vi "strip highlighting.vi"(0 "input string":string) -> (2 "Selection":bool, 3 "Selection cluster":cluster{i32, i32, "selected string":string}, 4 "output string":string, 6 "Highlighted string":string, 8 "Highlighting":bool, 10 "Line #":i32, 15 "error out":errorcluster)   [LabVIEW 2018]
uses:
  <vilib>/regexp/Match Regular Expression.xnode
panel:
  out "whole match":string
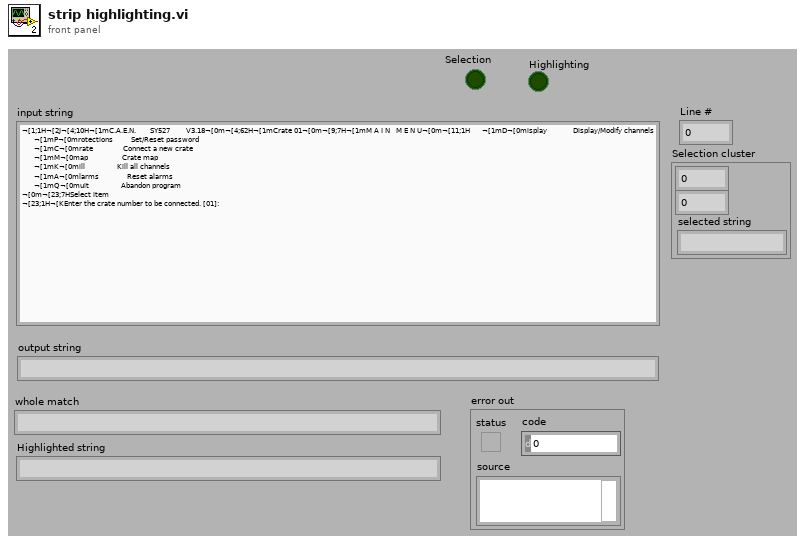
[diagram p1: front panel]
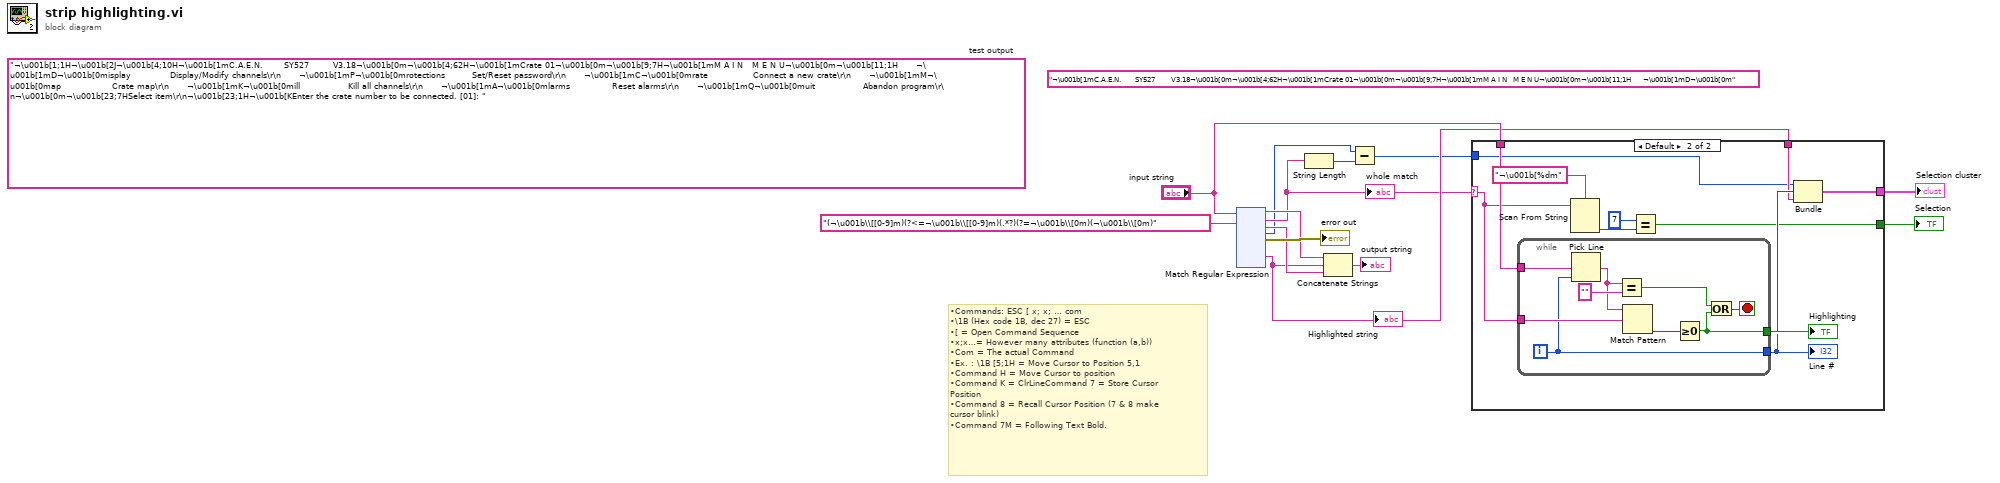
[diagram p0: block diagram]
diagram:
  (unwired) "¬\u001b[1mC.A.E.N.       SY527        V3.18¬\u001b[0m¬\u001b[4;62H¬\u001b[1mCrate 01¬\u001b[0m¬\u001b[9;7H¬\u001b[1mM A I N   M E N U¬\u001b[0m¬\u001b[11;1H      ¬\u001b[1mD¬\u001b[0m" ("whole match 2")
  (unwired) "¬\u001b[1;1H¬\u001b[2J¬\u001b[4;10H¬\u001b[1mC.A.E.N.       SY527        V3.18¬\u001b[0m¬\u001b[4;62H¬\u001b[1mCrate 01¬\u001b[0m¬\u001b[9;7H¬\u001b[1mM A I N   M E N U¬\u001b[0m¬\u001b[11;1H      ¬\u001b[1mD¬\u001b[0misplay             Display/Modify channels\r\n      ¬\u001b[1mP¬\u001b[0mrotections         Set/Reset password\r\n      ¬\u001b[1mC¬\u001b[0mrate               Connect a new crate\r\n      ¬\u001b[1mM¬\u001b[0map                 Crate map\r\n      ¬\u001b[1mK¬\u001b[0mill                Kill all channels\r\n      ¬\u001b[1mA¬\u001b[0mlarms              Reset alarms\r\n      ¬\u001b[1mQ¬\u001b[0muit                Abandon program\r\n¬\u001b[0m¬\u001b[23;7HSelect item\r\n¬\u001b[23;1H¬\u001b[KEnter the crate number to be connected. [01]: "  # test output
  # "•Commands: ESC [ x; x; … com \n•\\1B (Hex code 1B, dec 27) = ESC \n•[ = Open Command Sequence \n•x;x…= However many attributes (function (a,b)) \n•Com = The actual Command \n•Ex. : \\1B [5;1H = Move Cursor to Position 5,1 \n•Command H = Move Cursor to position \n•Command K = ClrLineCommand 7 = Store Cursor \nPosition \n•Command 8 = Recall Cursor Position (7 & 8 make \ncursor blink) \n•Command 7M = Following Text Bold."
  n1 = xnode "Match Regular Expression"("input string"="input string", "regular expression"="(¬\u001b\\[[0-9]m)(?<=¬\u001b\\[[0-9]m)(.*?)(?=¬\u001b\\[0m)(¬\u001b\\[0m)" ("search string")) -> ("before match"=w11:string, "whole match"=w3:string, "after match"=w10:string, "offset past match"=w2:i32, "error out"=→"error out":errorcluster, "submatch 2"=w5:string)  [unwired: 4 in, 2 out]
  "whole match" <- w3
  "Highlighted string" <- w5
  n2 = String Length(string=w3) -> (length=w4:i32)
  n3 = Concatenate Strings(w11, w5, w10) -> (→"output string":string)
  n4 = Subtract(x=w2, y=w4) -> (x-y=w1:i32)
  n5 = case shown="Default" w3 {
    selector: w3 -> [_ w19]
    tunnel: "input string" -> [_ w24]
    tunnel: [_ w17] -> w7
    tunnel: [_ w16] -> w6
    tunnel: w5 -> [_ w15]
    tunnel: w1 -> [_ w14]
    frame "" {
    }
    frame Default {
      n6 = while {
        tunnel: w24 -> [w33]
        tunnel: w19 -> [w29]
        tunnel: [w27] -> w18
        tunnel: [w26] -> w23
        i -> [w27]
        stop <- w28 stop-if-true
        n7 = Pick Line(multi-line string=w33, line index=w27) -> (output string=w30:string)  [unwired: 1 in]
        n8 = Equal?(x=w30, y="") -> (x = y?=w31:bool)
        n9 = Match Pattern(string=w30, regular expression=w29) -> (offset past match=w25:i32)  [unwired: 1 in, 3 out]
        n10 = Greater Or Equal To 0?(x=w25) -> (x >= 0?=w26:bool)
        n11 = Or(x=w31, y=w26) -> (x .or. y?=w28:bool)
      }
      "Line #" <- w18
      "Highlighting" <- w23
      n12 = Scan From String(format string="¬\u001b[%dm", input string=w19) -> (output 1=w21:i32)  [unwired: 3 in, 3 out]
      n13 = Equal?(x=7, y=w21) -> (x = y?=w17:bool)
      n14 = Bundle(w14, w18, "submatch 2"=w15) -> (w16:cluster{i32, i32, "submatch 2":string})  [unwired: 1 in]
    }
  }
  "Selection" <- w7
  "Selection cluster" <- w6
